vi "Disconnect UDP.vi"(8 "error in (no error)":errorcluster, 11 "Telnet V2 in":refnum<class "Telnet V2.lvclass">) -> (0 "error out":errorcluster, 3 "Telnet V2 out":refnum<class "Telnet V2.lvclass">)   [LabVIEW 2018, in "Telnet V2.lvlib" / "Telnet V2.lvclass"]
uses:
  Telnet V2.lvclass
  Telnet V2.lvclass/Telnet V2.ctl
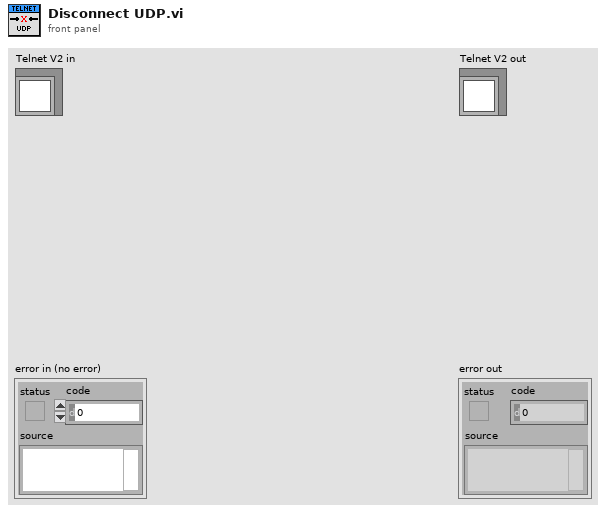
[diagram p1: front panel]
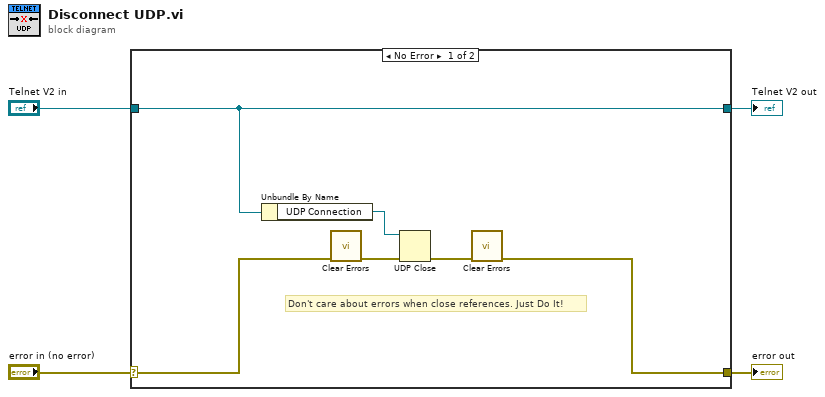
[diagram p0: block diagram]
diagram:
  n1 = case shown="No Error" "error in (no error)" {
    selector: "error in (no error)" -> [w9 w12]
    tunnel: [w8 w12] -> w3
    tunnel: [w10 w11] -> w1
    tunnel: "Telnet V2 in" -> [w10 w11]
    frame No Error {
      # "Don't care about errors when close references. Just Do It!"
      n2 = Unbundle By Name(w10) -> ("UDP Connection"=w5:refnum<k16>)
      n3 = call <vilib>:"Clear Errors.vi"("error in (no error)"=w9) -> ("error out"=w7:errorcluster)  [unwired: 5 in, 1 out]
      n4 = UDP Close(connection ID=w5, 8:w7) -> (error out=w6:errorcluster)  [unwired: 1 out]
      n5 = call <vilib>:"Clear Errors.vi"("error in (no error)"=w6) -> ("error out"=w8:errorcluster)  [unwired: 5 in, 1 out]
    }
    frame Error {
    }
  }
  "error out" <- w3
  "Telnet V2 out" <- w1
